vi "Begin.vi"(8 "error in":errorcluster) -> (0 "error out":errorcluster)   [LabVIEW 2017]
doc: "Called before other user functions, this VI is expected to open initial I/O refnums, load in file data, and do all program initialization. Notice that the <B>error out</B> terminal is simply used for data flow. Wiring it to other structures or subVIs ensures that this VI runs first."
uses:
  <vilib>/Rock Robotics/WPI/DriverStation/WPI_DriverStationRobotMode2.ctl
  <vilib>/Rock Robotics/WPI/Joystick/WPI_JoystickDeviceEnum.ctl
  Robot Global Data.vi
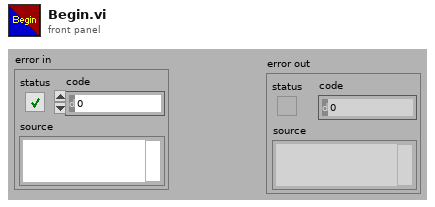
[diagram p1: front panel]
types:
  T1 = typedef "WPI_JoystickDeviceEnum.ctl" = enum16{"USB 0", "USB 1", "USB 2", "USB 3", "USB 4", "USB 5"}
  T2 = typedef "WPI_DriverStationRobotMode2.ctl" = enum16{"Autonomous Disabled", "Autonomous Enabled", "Teleop Disabled", "Teleop Enabled", "Disconnected", "Finish", "Test Disabled", "Test Enabled", "Emergency Stopped"}
  T3 = typedef "WPI_MotorControlDeviceRef.ctl" = cluster{"DeviceStatus":errorcluster, "Type":T4, "PWM":cluster{"PWM Channel":T5, "DeadBand":T6}, "CAN":cluster{"Device Number":u8, "SetOutput VI Ref":variant, "GetOutput VI Ref":variant, "Enable VI Ref":variant, "Disable VI Ref":variant, "Data":variant}, "Invert":bool, "DIO PWM":cluster{"PWM \"Enable\" Channel":T5, "DIOChannel":T7, "PWM Rate":dbl}}
  T4 = typedef "WPI_MotorControlType.ctl" = enum16{"PWM", "CAN", "DIO PWM"}
  T5 = typedef "FPGA_DIOPWMChannel.ctl" = enum8{"PWM 0", "PWM 1", "PWM 2", "PWM 3", "PWM 4", "PWM 5", "PWM 6", "PWM 7", "PWM 8", "PWM 9", "PWM MXP 0", "PWM MXP 1", "PWM MXP 2", "PWM MXP 3", "PWM MXP 4", "PWM MXP 5", "PWM MXP 6", "PWM MXP 7", "PWM MXP 8", "PWM MXP 9", "Invalid"}
  T6 = typedef "WPI_PWMDeadband.ctl" = cluster{"Name":string, "maxPositivePwm":i32, "minPositivePwm":i32, "centerPwm":i32, "maxNegativePwm":i32, "minNegativePwm":i32, "angularRange":u16}
  T7 = typedef "FPGA_DIOChannel.ctl" = enum8{"DIO 0", "DIO 1", "DIO 2", "DIO 3", "DIO 4", "DIO 5", "DIO 6", "DIO 7", "DIO 8", "DIO 9", "DIO MXP 0", "DIO MXP 1", "DIO MXP 2", "DIO MXP 3", "DIO MXP 4", "DIO MXP 5", "DIO MXP 6", "DIO MXP 7", "DIO MXP 8", "DIO MXP 9", "DIO MXP 10", "DIO MXP 11", "DIO MXP 12", "DIO MXP 13", "DIO MXP 14", "DIO MXP 15", "SPI Port CS1", "SPI Port CS2", "SPI Port CS3", "SPI Port MISO", "SPI Port MOSI", "Invalid"}
  T8 = typedef "WPI_JoystickDevRef.ctl" = cluster{"Device":T1}
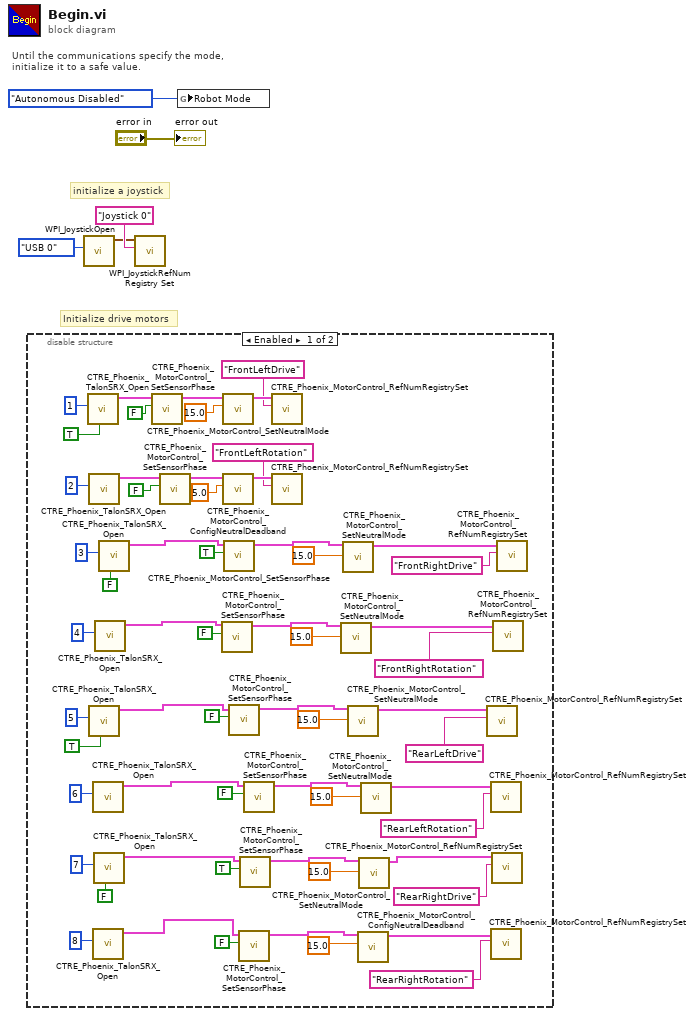
[diagram p0: block diagram]
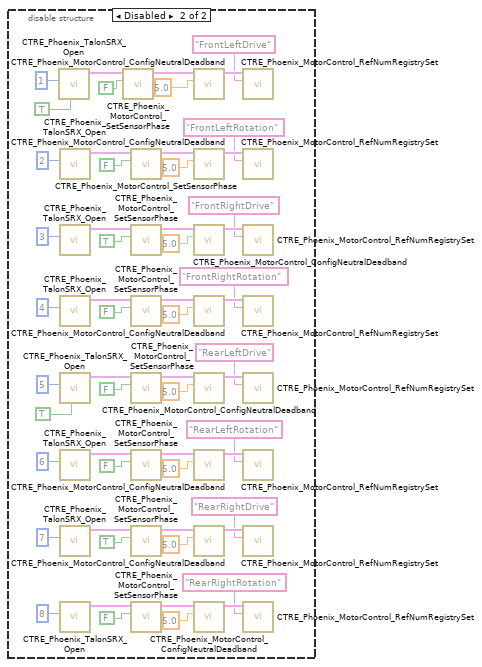
[diagram p2: hidden frame]
diagram:
  # "Initialize drive motors"
  # "initialize a joystick"
  # "Until the communications specify the mode,\ninitialize it to a safe value."
  n1 = disable-structure shown="Enabled" {
    frame Enabled {
      n2 = call "CTRE_Phoenix_TalonSRX_Open.vi"("Invert"=TRUE, "Device Number"=u8 1) -> ("CAN Talon SRX Ref"=w34:T3)  [unwired: 8 in, 1 out]
      n3 = call "CTRE_Phoenix_TalonSRX_Open.vi"("Device Number"=u8 2) -> ("CAN Talon SRX Ref"=w32:T3)  [unwired: 9 in, 1 out]
      n4 = call "CTRE_Phoenix_TalonSRX_Open.vi"("Invert"=TRUE, "Device Number"=u8 5) -> ("CAN Talon SRX Ref"=w26:T3)  [unwired: 8 in, 1 out]
      n5 = call "CTRE_Phoenix_TalonSRX_Open.vi"("Device Number"=u8 6) -> ("CAN Talon SRX Ref"=w24:T3)  [unwired: 9 in, 1 out]
      n6 = call "CTRE_Phoenix_TalonSRX_Open.vi"("Device Number"=u8 8) -> ("CAN Talon SRX Ref"=w20:T3)  [unwired: 9 in, 1 out]
      n7 = call "CTRE_Phoenix_TalonSRX_Open.vi"("Invert"=FALSE, "Device Number"=u8 7) -> ("CAN Talon SRX Ref"=w22:T3)  [unwired: 8 in, 1 out]
      n8 = call "CTRE_Phoenix_TalonSRX_Open.vi"("Device Number"=u8 4) -> ("CAN Talon SRX Ref"=w28:T3)  [unwired: 9 in, 1 out]
      n9 = call "CTRE_Phoenix_TalonSRX_Open.vi"("Invert"=FALSE, "Device Number"=u8 3) -> ("CAN Talon SRX Ref"=w30:T3)  [unwired: 8 in, 1 out]
      n10 = call "CTRE_Phoenix_MotorControl_SetSensorPhase.vi"("PhaseSensor"=FALSE, "PhoenixMotorControlDevRef"=w34) -> ("PhoenixMotorControlDevRef"=w43:T3)  [unwired: 8 in, 1 out]
      n11 = call "CTRE_Phoenix_MotorControl_SetSensorPhase.vi"("PhaseSensor"=FALSE, "PhoenixMotorControlDevRef"=w32) -> ("PhoenixMotorControlDevRef"=w42:T3)  [unwired: 8 in, 1 out]
      n12 = call "CTRE_Phoenix_MotorControl_SetSensorPhase.vi"("PhaseSensor"=FALSE, "PhoenixMotorControlDevRef"=w28) -> ("PhoenixMotorControlDevRef"=w40:T3)  [unwired: 8 in, 1 out]
      n13 = call "CTRE_Phoenix_MotorControl_SetNeutralMode.vi"("Motor Control Neutral Mode"=15.0, "PhoenixMotorControlDevRef"=w43) -> ("PhoenixMotorControlDevRef"=w33:T3)  [unwired: 8 in, 1 out]
      n14 = call "CTRE_Phoenix_MotorControl_ConfigNeutralDeadband.vi"("Percent Deadband"=5.0, "PhoenixMotorControlDevRef"=w42) -> ("PhoenixMotorControlDevRef"=w31:T3)  [unwired: 8 in, 1 out]
      n15 = call "CTRE_Phoenix_MotorControl_SetSensorPhase.vi"("PhaseSensor"=TRUE, "PhoenixMotorControlDevRef"=w30) -> ("PhoenixMotorControlDevRef"=w41:T3)  [unwired: 8 in, 1 out]
      n16 = call "CTRE_Phoenix_MotorControl_SetSensorPhase.vi"("PhaseSensor"=FALSE, "PhoenixMotorControlDevRef"=w26) -> ("PhoenixMotorControlDevRef"=w39:T3)  [unwired: 8 in, 1 out]
      n17 = call "CTRE_Phoenix_MotorControl_SetSensorPhase.vi"("PhaseSensor"=FALSE, "PhoenixMotorControlDevRef"=w20) -> ("PhoenixMotorControlDevRef"=w36:T3)  [unwired: 8 in, 1 out]
      n18 = call "CTRE_Phoenix_MotorControl_SetSensorPhase.vi"("PhaseSensor"=TRUE, "PhoenixMotorControlDevRef"=w22) -> ("PhoenixMotorControlDevRef"=w37:T3)  [unwired: 8 in, 1 out]
      n19 = call "CTRE_Phoenix_MotorControl_SetSensorPhase.vi"("PhaseSensor"=FALSE, "PhoenixMotorControlDevRef"=w24) -> ("PhoenixMotorControlDevRef"=w38:T3)  [unwired: 8 in, 1 out]
      n20 = call "CTRE_Phoenix_MotorControl_RefNumRegistrySet.vi"("refnum name"="FrontLeftDrive", "PhoenixMotorControlDevRef"=w33) -> ()  [unwired: 8 in, 2 out]
      n21 = call "CTRE_Phoenix_MotorControl_RefNumRegistrySet.vi"("refnum name"="FrontLeftRotation", "PhoenixMotorControlDevRef"=w31) -> ()  [unwired: 8 in, 2 out]
      n22 = call "CTRE_Phoenix_MotorControl_SetNeutralMode.vi"("Motor Control Neutral Mode"=15.0, "PhoenixMotorControlDevRef"=w40) -> ("PhoenixMotorControlDevRef"=w27:T3)  [unwired: 8 in, 1 out]
      n23 = call "CTRE_Phoenix_MotorControl_SetNeutralMode.vi"("Motor Control Neutral Mode"=15.0, "PhoenixMotorControlDevRef"=w41) -> ("PhoenixMotorControlDevRef"=w29:T3)  [unwired: 8 in, 1 out]
      n24 = call "CTRE_Phoenix_MotorControl_SetNeutralMode.vi"("Motor Control Neutral Mode"=15.0, "PhoenixMotorControlDevRef"=w39) -> ("PhoenixMotorControlDevRef"=w25:T3)  [unwired: 8 in, 1 out]
      n25 = call "CTRE_Phoenix_MotorControl_ConfigNeutralDeadband.vi"("Percent Deadband"=15.0, "PhoenixMotorControlDevRef"=w36) -> ("PhoenixMotorControlDevRef"=w19:T3)  [unwired: 8 in, 1 out]
      n26 = call "CTRE_Phoenix_MotorControl_SetNeutralMode.vi"("Motor Control Neutral Mode"=15.0, "PhoenixMotorControlDevRef"=w37) -> ("PhoenixMotorControlDevRef"=w21:T3)  [unwired: 8 in, 1 out]
      n27 = call "CTRE_Phoenix_MotorControl_SetNeutralMode.vi"("Motor Control Neutral Mode"=15.0, "PhoenixMotorControlDevRef"=w38) -> ("PhoenixMotorControlDevRef"=w23:T3)  [unwired: 8 in, 1 out]
      n28 = call "CTRE_Phoenix_MotorControl_RefNumRegistrySet.vi"("refnum name"="RearLeftDrive", "PhoenixMotorControlDevRef"=w25) -> ()  [unwired: 8 in, 2 out]
      n29 = call "CTRE_Phoenix_MotorControl_RefNumRegistrySet.vi"("refnum name"="RearLeftRotation", "PhoenixMotorControlDevRef"=w23) -> ()  [unwired: 8 in, 2 out]
      n30 = call "CTRE_Phoenix_MotorControl_RefNumRegistrySet.vi"("refnum name"="RearRightRotation", "PhoenixMotorControlDevRef"=w19) -> ()  [unwired: 8 in, 2 out]
      n31 = call "CTRE_Phoenix_MotorControl_RefNumRegistrySet.vi"("refnum name"="RearRightDrive", "PhoenixMotorControlDevRef"=w21) -> ()  [unwired: 8 in, 2 out]
      n32 = call "CTRE_Phoenix_MotorControl_RefNumRegistrySet.vi"("refnum name"="FrontRightRotation", "PhoenixMotorControlDevRef"=w27) -> ()  [unwired: 8 in, 2 out]
      n33 = call "CTRE_Phoenix_MotorControl_RefNumRegistrySet.vi"("refnum name"="FrontRightDrive", "PhoenixMotorControlDevRef"=w29) -> ()  [unwired: 8 in, 2 out]
    }
    frame Disabled {
      n34 = call "CTRE_Phoenix_TalonSRX_Open.vi"("Invert"=TRUE, "Device Number"=u8 1) -> ("CAN Talon SRX Ref"=w117:T3)  [unwired: 8 in, 1 out]
      n35 = call "CTRE_Phoenix_TalonSRX_Open.vi"("Device Number"=u8 2) -> ("CAN Talon SRX Ref"=w115:T3)  [unwired: 9 in, 1 out]
      n36 = call "CTRE_Phoenix_TalonSRX_Open.vi"("Device Number"=u8 3) -> ("CAN Talon SRX Ref"=w106:T3)  [unwired: 9 in, 1 out]
      n37 = call "CTRE_Phoenix_TalonSRX_Open.vi"("Device Number"=u8 4) -> ("CAN Talon SRX Ref"=w100:T3)  [unwired: 9 in, 1 out]
      n38 = call "CTRE_Phoenix_TalonSRX_Open.vi"("Invert"=TRUE, "Device Number"=u8 5) -> ("CAN Talon SRX Ref"=w93:T3)  [unwired: 8 in, 1 out]
      n39 = call "CTRE_Phoenix_TalonSRX_Open.vi"("Device Number"=u8 6) -> ("CAN Talon SRX Ref"=w87:T3)  [unwired: 9 in, 1 out]
      n40 = call "CTRE_Phoenix_TalonSRX_Open.vi"("Device Number"=u8 7) -> ("CAN Talon SRX Ref"=w82:T3)  [unwired: 9 in, 1 out]
      n41 = call "CTRE_Phoenix_TalonSRX_Open.vi"("Device Number"=u8 8) -> ("CAN Talon SRX Ref"=w75:T3)  [unwired: 9 in, 1 out]
      n42 = call "CTRE_Phoenix_MotorControl_SetSensorPhase.vi"("PhaseSensor"=FALSE, "PhoenixMotorControlDevRef"=w117) -> ("PhoenixMotorControlDevRef"=w119:T3)  [unwired: 8 in, 1 out]
      n43 = call "CTRE_Phoenix_MotorControl_SetSensorPhase.vi"("PhaseSensor"=FALSE, "PhoenixMotorControlDevRef"=w115) -> ("PhoenixMotorControlDevRef"=w118:T3)  [unwired: 8 in, 1 out]
      n44 = call "CTRE_Phoenix_MotorControl_SetSensorPhase.vi"("PhaseSensor"=TRUE, "PhoenixMotorControlDevRef"=w106) -> ("PhoenixMotorControlDevRef"=w105:T3)  [unwired: 8 in, 1 out]
      n45 = call "CTRE_Phoenix_MotorControl_SetSensorPhase.vi"("PhaseSensor"=FALSE, "PhoenixMotorControlDevRef"=w100) -> ("PhoenixMotorControlDevRef"=w99:T3)  [unwired: 8 in, 1 out]
      n46 = call "CTRE_Phoenix_MotorControl_SetSensorPhase.vi"("PhaseSensor"=FALSE, "PhoenixMotorControlDevRef"=w93) -> ("PhoenixMotorControlDevRef"=w94:T3)  [unwired: 8 in, 1 out]
      n47 = call "CTRE_Phoenix_MotorControl_SetSensorPhase.vi"("PhaseSensor"=FALSE, "PhoenixMotorControlDevRef"=w87) -> ("PhoenixMotorControlDevRef"=w88:T3)  [unwired: 8 in, 1 out]
      n48 = call "CTRE_Phoenix_MotorControl_SetSensorPhase.vi"("PhaseSensor"=TRUE, "PhoenixMotorControlDevRef"=w82) -> ("PhoenixMotorControlDevRef"=w81:T3)  [unwired: 8 in, 1 out]
      n49 = call "CTRE_Phoenix_MotorControl_SetSensorPhase.vi"("PhaseSensor"=FALSE, "PhoenixMotorControlDevRef"=w75) -> ("PhoenixMotorControlDevRef"=w76:T3)  [unwired: 8 in, 1 out]
      n50 = call "CTRE_Phoenix_MotorControl_ConfigNeutralDeadband.vi"("Percent Deadband"=5.0, "PhoenixMotorControlDevRef"=w119) -> ("PhoenixMotorControlDevRef"=w116:T3)  [unwired: 8 in, 1 out]
      n51 = call "CTRE_Phoenix_MotorControl_ConfigNeutralDeadband.vi"("Percent Deadband"=5.0, "PhoenixMotorControlDevRef"=w118) -> ("PhoenixMotorControlDevRef"=w114:T3)  [unwired: 8 in, 1 out]
      n52 = call "CTRE_Phoenix_MotorControl_ConfigNeutralDeadband.vi"("Percent Deadband"=5.0, "PhoenixMotorControlDevRef"=w105) -> ("PhoenixMotorControlDevRef"=w107:T3)  [unwired: 8 in, 1 out]
      n53 = call "CTRE_Phoenix_MotorControl_ConfigNeutralDeadband.vi"("Percent Deadband"=5.0, "PhoenixMotorControlDevRef"=w99) -> ("PhoenixMotorControlDevRef"=w101:T3)  [unwired: 8 in, 1 out]
      n54 = call "CTRE_Phoenix_MotorControl_ConfigNeutralDeadband.vi"("Percent Deadband"=5.0, "PhoenixMotorControlDevRef"=w94) -> ("PhoenixMotorControlDevRef"=w92:T3)  [unwired: 8 in, 1 out]
      n55 = call "CTRE_Phoenix_MotorControl_ConfigNeutralDeadband.vi"("Percent Deadband"=5.0, "PhoenixMotorControlDevRef"=w88) -> ("PhoenixMotorControlDevRef"=w86:T3)  [unwired: 8 in, 1 out]
      n56 = call "CTRE_Phoenix_MotorControl_ConfigNeutralDeadband.vi"("Percent Deadband"=5.0, "PhoenixMotorControlDevRef"=w81) -> ("PhoenixMotorControlDevRef"=w83:T3)  [unwired: 8 in, 1 out]
      n57 = call "CTRE_Phoenix_MotorControl_ConfigNeutralDeadband.vi"("Percent Deadband"=5.0, "PhoenixMotorControlDevRef"=w76) -> ("PhoenixMotorControlDevRef"=w74:T3)  [unwired: 8 in, 1 out]
      n58 = call "CTRE_Phoenix_MotorControl_RefNumRegistrySet.vi"("refnum name"="FrontLeftDrive", "PhoenixMotorControlDevRef"=w116) -> ()  [unwired: 8 in, 2 out]
      n59 = call "CTRE_Phoenix_MotorControl_RefNumRegistrySet.vi"("refnum name"="FrontLeftRotation", "PhoenixMotorControlDevRef"=w114) -> ()  [unwired: 8 in, 2 out]
      n60 = call "CTRE_Phoenix_MotorControl_RefNumRegistrySet.vi"("refnum name"="FrontRightDrive", "PhoenixMotorControlDevRef"=w107) -> ()  [unwired: 8 in, 2 out]
      n61 = call "CTRE_Phoenix_MotorControl_RefNumRegistrySet.vi"("refnum name"="FrontRightRotation", "PhoenixMotorControlDevRef"=w101) -> ()  [unwired: 8 in, 2 out]
      n62 = call "CTRE_Phoenix_MotorControl_RefNumRegistrySet.vi"("refnum name"="RearLeftDrive", "PhoenixMotorControlDevRef"=w92) -> ()  [unwired: 8 in, 2 out]
      n63 = call "CTRE_Phoenix_MotorControl_RefNumRegistrySet.vi"("refnum name"="RearLeftRotation", "PhoenixMotorControlDevRef"=w86) -> ()  [unwired: 8 in, 2 out]
      n64 = call "CTRE_Phoenix_MotorControl_RefNumRegistrySet.vi"("refnum name"="RearRightDrive", "PhoenixMotorControlDevRef"=w83) -> ()  [unwired: 8 in, 2 out]
      n65 = call "CTRE_Phoenix_MotorControl_RefNumRegistrySet.vi"("refnum name"="RearRightRotation", "PhoenixMotorControlDevRef"=w74) -> ()  [unwired: 8 in, 2 out]
    }
  }
  n66 = call <vilib>:"WPI_JoystickOpen.vi"("JoystickDevice"=WPI_JoystickDeviceEnum."USB 0") -> ("JoystickDevRef"=w3:T8)  [unwired: 10 in]
  n67 = call <vilib>:"WPI_JoystickRefNum Registry Set.vi"("refnum name"="Joystick 0", "JoystickDevRef"=w3) -> ()  [unwired: 8 in, 2 out]
  n68 = global write "Robot Global Data.vi" "Robot Mode"(WPI_DriverStationRobotMode2."Autonomous Disabled" ("Robot Mode")) -> ()
  "error out" <- "error in"
